vi "FTW-JSON-LexicalScan-Unget.vi"(0 "JSON String":T1, 11 "error in":errorcluster) -> (4 "JSON String Out":T1, 8 "Char":u8, 15 "error out":errorcluster)   [LabVIEW 2015]
uses:
  FTW-JSON-LexicalScan.ctl
panel:
  # "Inputs"
  # "Outputs"
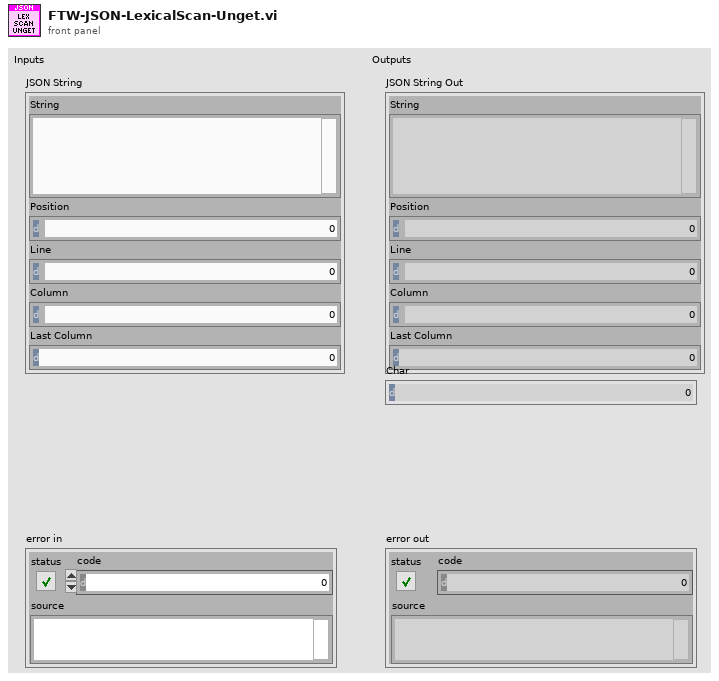
[diagram p1: front panel]
types:
  T1 = typedef "FTW-JSON-LexicalScan.ctl" = cluster{"String":string, "Position":i32, "Line":i32, "Column":i32, "Last Column":i32}
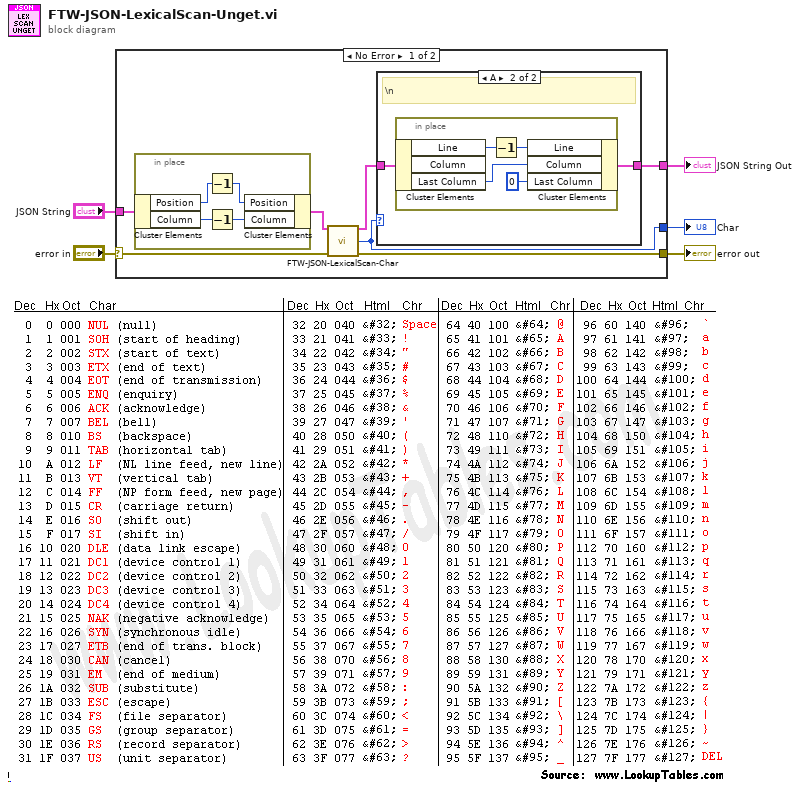
[diagram p0: block diagram]
diagram:
  n1 = case shown="No Error" "error in" {
    selector: "error in" -> [w12 w24]
    tunnel: "JSON String" -> [w11 w25]
    tunnel: [w10 w24] -> w3
    tunnel: [w7 w25] -> w2
    tunnel: [w6 _] -> w1
    frame No Error {
      n2 = in-place {
        n3 = in-place-cluster #1(w11) -> ("Position"=w23:i32, "Column"=w21:i32)
        n4 = Decrement(x=w23) -> (x-1=w22:i32)
        n5 = Decrement(x=w21) -> (x-1=w20:i32)
        n6 = in-place-cluster #1("Position"=w22, "Column"=w20) -> (w9:T1)
      }
      n7 = call "FTW-JSON-LexicalScan-Char.vi"("JSON String"=w9, "error in"=w12) -> ("JSON String Out"=w8:T1, "Char"=w6:u8, "error out"=w10:errorcluster)  [unwired: 11 in]
      n8 = case shown="A" w6 {
        tunnel: w8 -> [w13 w15]
        tunnel: [w13 w14] -> w7
        frame 0, Default {
        }
        frame 10 {
          # "\\n"
          n9 = in-place {
            n10 = in-place-cluster #2(w15) -> ("Line"=w19:i32, "Last Column"=w17:i32)  [unwired: 1 out]
            n11 = Decrement(x=w19) -> (x-1=w18:i32)
            n12 = in-place-cluster #2("Line"=w18, "Column"=w17, "Last Column"=0) -> (w14:T1)
          }
        }
      }
    }
    frame Error {
    }
  }
  "error out" <- w3
  "JSON String Out" <- w2
  "Char" <- w1
